vi "Drive Controller.vi"(8 "error in":errorcluster) -> ()   [LabVIEW 2019]
doc: "This VI executes continuously carrying out the current operation and responding to updates or new operation requests. It will often contain the timing or control code that is difficult to place directly in TeleOp. This VI generally opens all sensors and motors and isolates the rest of the robot code from knowing implementation details of how the operations are carried out."
uses:
  <vilib>/Rock Robotics/WPI/Framework/Completion Status.ctl
  Drive Setpoints.ctl
  Drive Operations.ctl
  <vilib>/Rock Robotics/WPI/SafetyOutput/WPI_SafetyOutputConfigMenu.ctl
  <vilib>/Rock Robotics/WPI/RobotDrive/WPI_RobotDriveOpen4MotorWithExistingMotors.vi
  <vilib>/Rock Robotics/WPI/RobotDrive/WPI_RobotDriveOpen2MotorWithTalon.vi
panel:
  in  "Interactive Values":T1
  in  "Buttons":cluster{"Execute Cmd":bool, "Abort Cmd":bool}
  out "Command Timing":cluster{"Start Time (ms)":u32, "Iterations":i32}
  out "Status":T3
  out "Setpoints":T4(graph)
  out "Current\nCmd":string
  # "Tip: The graph shows the motor setpoints. It may also be helpful to observe inputs and sensor values.\nYou may also want to display tuning or debugging controls."
  # "Interactive Command: You may fill in the settings for a command\nand schedule it with the Execute button. You can observe and abort\nany command while fine tuning the code for the controller."
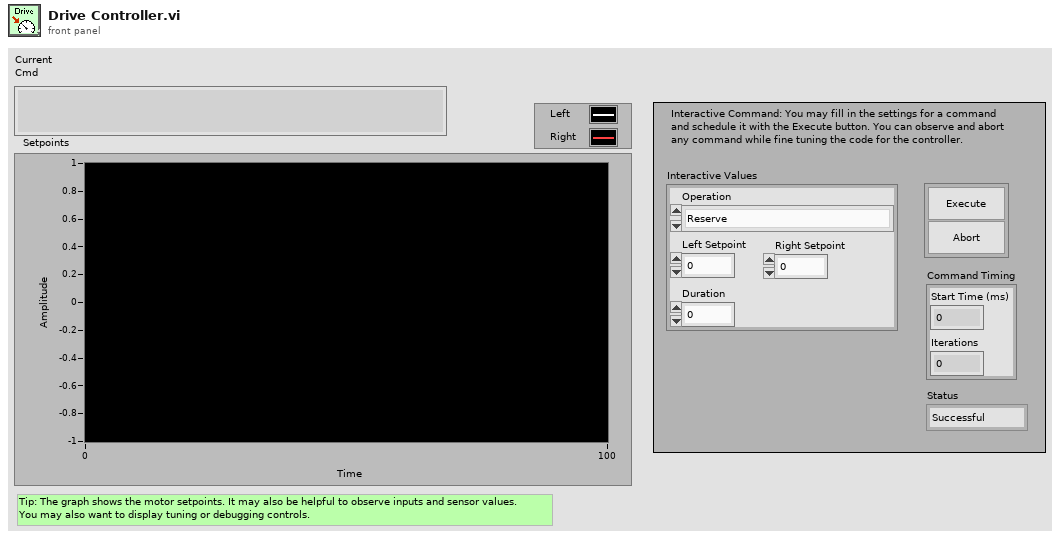
[diagram p1: front panel]
types:
  T1 = typedef "Drive Setpoints.ctl" = cluster{"Operation":T2, "Left Setpoint":dbl, "Right Setpoint":dbl, "Duration":dbl}
  T2 = typedef "Drive Operations.ctl" = enum16{"Reserve", "Read Current", "Immediate", "Drive for Time", "Drive for Distance"}
  T3 = typedef "Completion Status.ctl" = enum16{"Successful", "Aborted", "Incomplete"}
  T4 = cluster{"Left Setpoint":dbl, "Right Setpoint":dbl}
  T5 = typedef "WPI_SafetyOutputConfigMenu.ctl" = enum16{"Enable", "Disable"}
  T6 = typedef "WPI_RobotDriveDevRef.ctl" = cluster{"DevStatus":errorcluster, "Motors[]":T7[], "Square Inputs":bool, "Max Output":dbl}
  T7 = typedef "WPI_MotorControlDeviceRef.ctl" = cluster{"DeviceStatus":errorcluster, "Type":T8, "PWM":cluster{"PWM Channel":T9, "DeadBand":T10}, "CAN":cluster{"Device Number":u8, "SetOutput VI Ref":variant, "GetOutput VI Ref":variant, "Enable VI Ref":variant, "Disable VI Ref":variant, "Data":variant}, "Invert":bool, "DIO PWM":cluster{"PWM \"Enable\" Channel":T9, "DIOChannel":T11, "PWM Rate":dbl}}
  T8 = typedef "WPI_MotorControlType.ctl" = enum16{"PWM", "CAN", "DIO PWM"}
  T9 = typedef "FPGA_DIOPWMChannel.ctl" = enum8{"PWM 0", "PWM 1", "PWM 2", "PWM 3", "PWM 4", "PWM 5", "PWM 6", "PWM 7", "PWM 8", "PWM 9", "PWM MXP 0", "PWM MXP 1", "PWM MXP 2", "PWM MXP 3", "PWM MXP 4", "PWM MXP 5", "PWM MXP 6", "PWM MXP 7", "PWM MXP 8", "PWM MXP 9", "Invalid"}
  T10 = typedef "WPI_PWMDeadband.ctl" = cluster{"Name":string, "maxPositivePwm":i32, "minPositivePwm":i32, "centerPwm":i32, "maxNegativePwm":i32, "minNegativePwm":i32, "angularRange":u16}
  T11 = typedef "FPGA_DIOChannel.ctl" = enum8{"DIO 0", "DIO 1", "DIO 2", "DIO 3", "DIO 4", "DIO 5", "DIO 6", "DIO 7", "DIO 8", "DIO 9", "DIO MXP 0", "DIO MXP 1", "DIO MXP 2", "DIO MXP 3", "DIO MXP 4", "DIO MXP 5", "DIO MXP 6", "DIO MXP 7", "DIO MXP 8", "DIO MXP 9", "DIO MXP 10", "DIO MXP 11", "DIO MXP 12", "DIO MXP 13", "DIO MXP 14", "DIO MXP 15", "SPI Port CS1", "SPI Port CS2", "SPI Port CS3", "SPI Port MISO", "SPI Port MOSI", "Invalid"}
  T12 = typedef "Command Status Info.ctl" = cluster{"Name":string, "Status":T3, "notifier out":T13}
  T13 = typedef "Completion Notifier.ctl" = refnum<notifier>
  T14 = cluster{"SubSystem Data":T1, cluster{"Start Time (ms)":u32, "Iterations":i32}, cluster{"Command Info":T12, "Description":string, "Default Command":T1, "queue out":refnum<queue>, "Subsystem Name":string}}
  T15 = cluster{"SubSystem Data":T1, cluster{"Start Time (ms)":u32, "Iterations":i32}, "Default Command Arguments":cluster{"Command Info":T12, "Description":string, "Default Command":T1, "queue out":refnum<queue>, "Subsystem Name":string}}
  T16 = cluster{"Don't move motors while reserved":dbl, "Don't move motors while reserved":dbl}
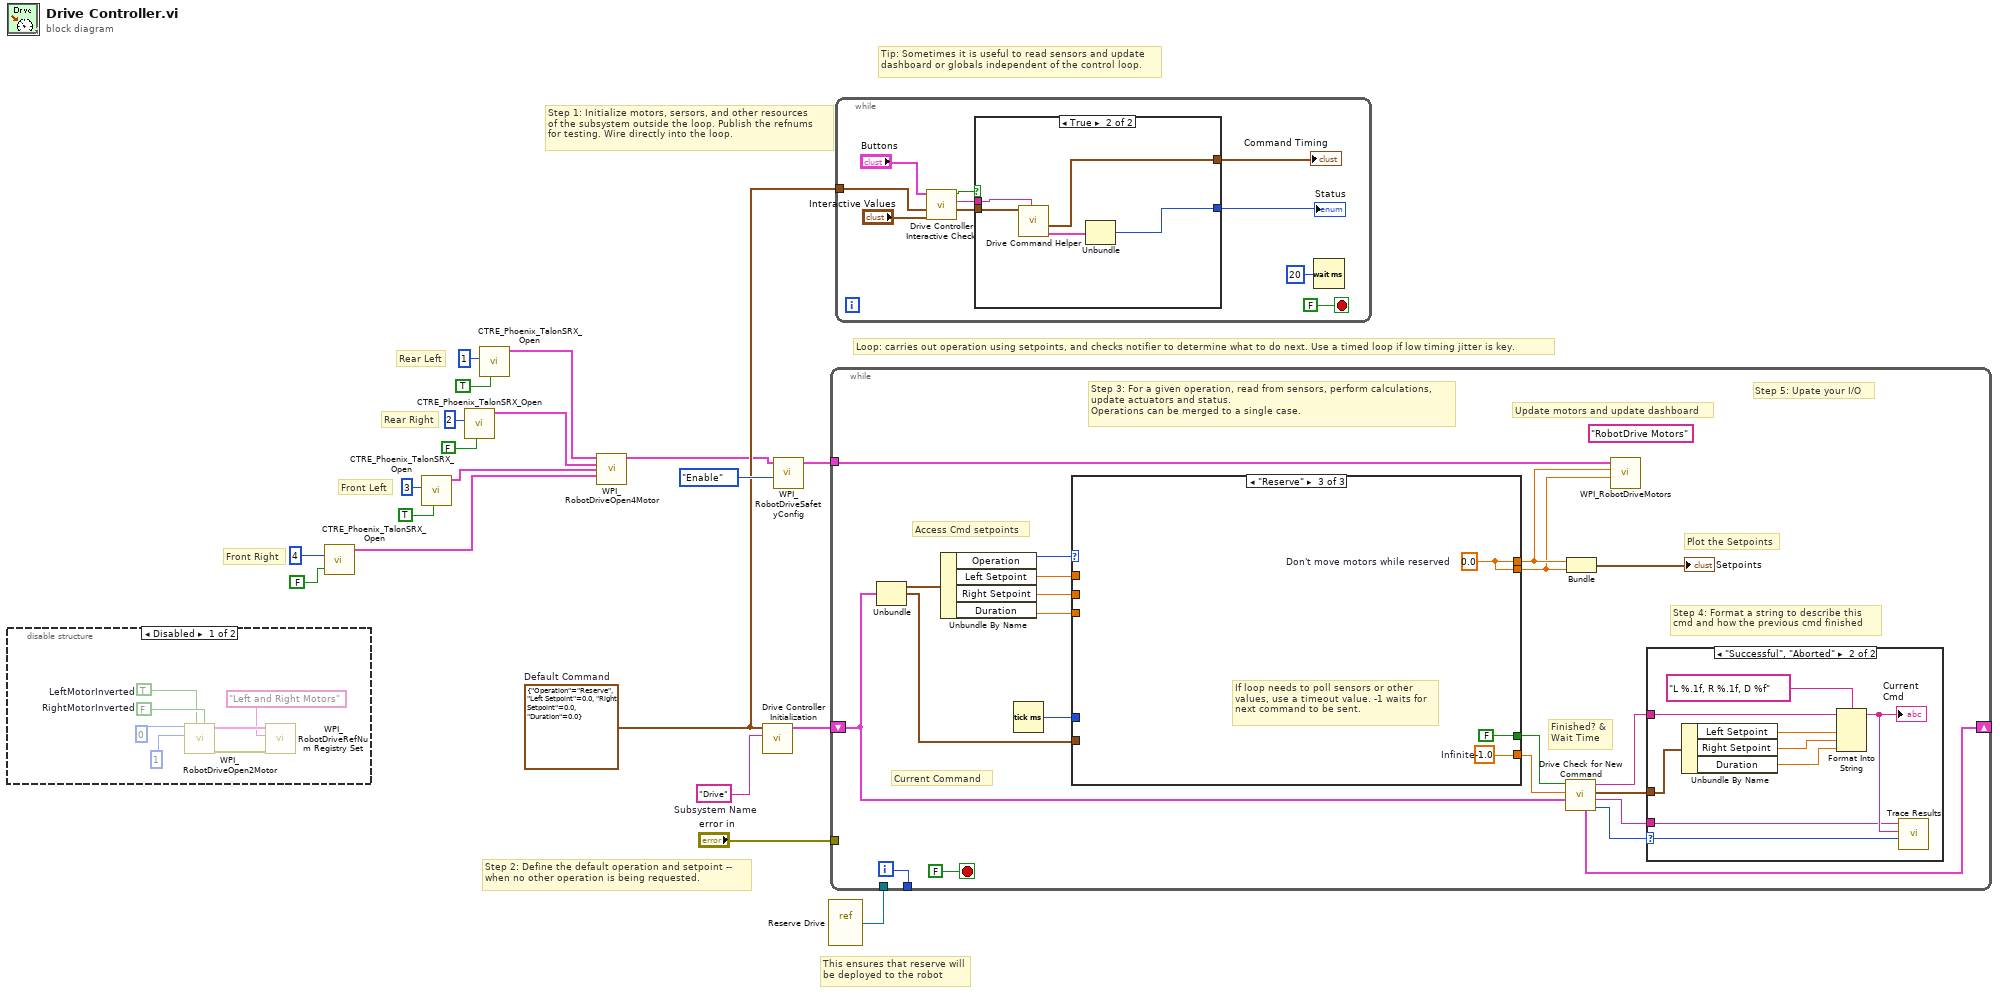
[diagram p0: block diagram]
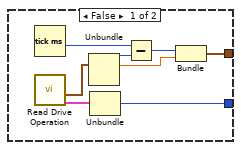
[diagram p3: hidden frame]
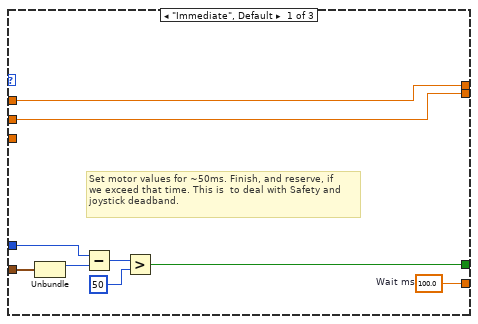
[diagram p5: hidden frame]
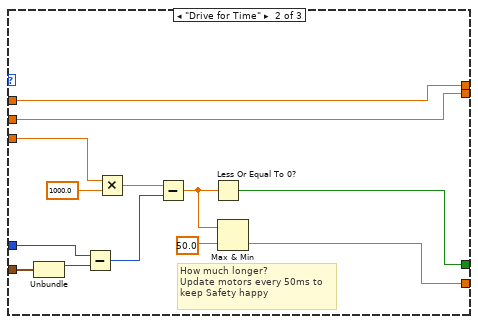
[diagram p6: hidden frame]
diagram:
  w14 = T1 {"Operation"=enum."Reserve", "Left Setpoint"=0.0, "Right Setpoint"=0.0, "Duration"=0.0}  # Default Command
  w20 = "Drive"  # Subsystem Name
  # "Front Right"
  # "Front Left"
  # "Rear Right"
  # "Rear Left"
  # "This ensures that reserve will\nbe deployed to the robot"
  # "Tip: Sometimes it is useful to read sensors and update\ndashboard or globals independent of the control loop."
  # "Step 2: Define the default operation and setpoint --\nwhen no other operation is being requested."
  # "Step 1: Initialize motors, sersors, and other resources\nof the subsystem outside the loop. Publish the refnums\nfor testing. Wire directly into the loop."
  # "Loop: carries out operation using setpoints, and checks notifier to determine what to do next. Use a timed loop if low timing jitter is key."
  n1 = disable-structure shown="Disabled" {
    frame Disabled {
      w24 = TRUE  # LeftMotorInverted
      w25 = FALSE  # RightMotorInverted
      n2 = call-poly <vilib>:"WPI_RobotDriveOpen2Motor.vi"("Right Motor Inverted"=w25, "Left Motor Inverted"=w24, "Right Motor"=u8 1 ("Left Motor"), "Left Motor"=u8 0) -> ("error out"=w21:errorcluster, "RobotDriveDevRef"=w23:T6)  [unwired: 1 in, 5 out]
      n3 = call <vilib>:"WPI_RobotDriveRefNum Registry Set.vi"("error in (no error)"=w21, "refnum name"="Left and Right Motors", "RobotDriveDevRef"=w23) -> ()  [unwired: 1 in, 8 out]
    }
    frame Enabled {
    }
  }
  n4 = call <vilib>:"CTRE_Phoenix_TalonSRX_Open.vi"("Invert"=FALSE, "Device Number"=u8 4) -> ("CAN Talon SRX Ref"=w2:T7)  [unwired: 8 in, 1 out]
  n5 = call <vilib>:"CTRE_Phoenix_TalonSRX_Open.vi"("Invert"=TRUE, "Device Number"=u8 3) -> ("CAN Talon SRX Ref"=w3:T7)  [unwired: 8 in, 1 out]
  n6 = call <vilib>:"CTRE_Phoenix_TalonSRX_Open.vi"("Invert"=FALSE, "Device Number"=u8 2) -> ("CAN Talon SRX Ref"=w4:T7)  [unwired: 8 in, 1 out]
  n7 = call <vilib>:"CTRE_Phoenix_TalonSRX_Open.vi"("Invert"=TRUE, "Device Number"=u8 1) -> ("CAN Talon SRX Ref"=w5:T7)  [unwired: 8 in, 1 out]
  n8 = call-poly <vilib>:"WPI_RobotDriveOpen4Motor.vi"("Rear Left Motor Dev Ref"=w5, "Rear Right Motor Dev Ref"=w4, "Front Left Motor Dev Ref"=w3, "Front Right Motor Dev Ref"=w2) -> ("RobotDriveDevRef"=w1:T6)  [unwired: 10 in, 1 out]
  n9 = call "Drive Controller Initialization.vi"("Subsystem Name"=w20, "Default Command"=w14) -> ("Current Command"=w16:T14)  [unwired: 9 in]
  n10 = call <vilib>:"WPI_RobotDriveSafetyConfig.vi"("mode"=WPI_SafetyOutputConfigMenu."Enable", "RobotDriveDevRef"=w1) -> ("RobotDriveDevRef"=w18:T6)  [unwired: 8 in, 1 out]
  n11 = vi-ref "Reserve Drive.vi"() -> (w15:refnum<vi>)
  n12 = while {
    shift-right: [w35] -> _
    shift-left: w16 -> [w28]
    tunnel: [w47] -> _
    tunnel: w18 -> [w43]
    tunnel: "error in" -> [_]
    tunnel: w15 -> [_]
    i -> [w47]
    stop <- FALSE stop-if-true
    (unwired) "RobotDrive Motors" ("Name")
    # "Step 5: Upate your I/O"
    # "Step 4: Format a string to describe this\ncmd and how the previous cmd finished"
    # "Current Command"
    # "Update motors and update dashboard"
    # "Plot the Setpoints"
    # "Access Cmd setpoints"
    # "Finished? &\nWait Time"
    # "Step 3: For a given operation, read from sensors, perform calculations,\nupdate actuators and status.\nOperations can be merged to a single case."
    n13 = Unbundle(w28) -> ("SubSystem Data"=w42:T1, w29:cluster{"Start Time (ms)":u32, "Iterations":i32})  [unwired: 1 out]
    n14 = Unbundle By Name(w42) -> ("Operation"=w41:T2, "Left Setpoint"=w40:dbl, "Right Setpoint"=w39:dbl, "Duration"=w38:dbl)
    n15 = Tick Count (ms)() -> (millisecond timer value=w37:u32)
    n16 = case shown="\"Reserve\"" w41 {
      tunnel: [w66 w67 w82] -> w34
      tunnel: [w59 w74 FALSE ("ignore previous (F)")] -> w33
      tunnel: w29 -> [w58 w76 _]
      tunnel: [w65 w73 w80] -> w45
      tunnel: [w64 w72 w80] -> w44
      tunnel: w40 -> [w65 w73 _]
      tunnel: w39 -> [w64 w72 _]
      tunnel: w38 -> [_ w71 _]
      tunnel: w37 -> [w60 w70 _]
      frame "Immediate", Default {
        w66 = 100.0  # Wait ms
        # "Set motor values for ~50ms. Finish, and reserve, if\nwe exceed that time. This is  to deal with Safety and\njoystick deadband."
        n17 = Unbundle(w58) -> ("Start Time (ms)"=w61:u32)  [unwired: 1 out]
        n18 = Subtract(x=w60, y=w61) -> (x-y=w62:u32)
        n19 = Greater?(x=w62, y=u8 50 ("Left Motor")) -> (0:w59:bool)
      }
      frame "Drive for Time" {
        # "How much longer?\nUpdate motors every 50ms to\nkeep Safety happy"
        n20 = Unbundle(w76) -> ("Start Time (ms)"=w75:u32)  [unwired: 1 out]
        n21 = Subtract(x=w70, y=w75) -> (x-y=w79:u32)
        n22 = Multiply(x=w71, y=1000.0) -> (x*y=w78:dbl)
        n23 = Subtract(x=w78, y=w79) -> (x-y=w69:dbl)
        n24 = Less Or Equal To 0?(x=w69) -> (x <= 0?=w74:bool)
        n25 = Max & Min(x=w69, y=50.0) -> (min(x,y)=w67:dbl)  [unwired: 1 out]
      }
      frame "Reserve" {
        w80 = 0.0  # Don't move motors while reserved
        w82 = -1.0  # Infinite
        # "If loop needs to poll sensors or other\nvalues, use a timeout value. -1 waits for\nnext command to be sent."
      }
    }
    n26 = call "Drive Check for New Command.vi"("input cluster"=w28, "Wait time (ms)"=w34, "Finished?"=w33) -> ("Completion"=w36:T3, "Subsystem Name"=w30:string, "Current Command"=w31:T1, "Initial Trace String"=w32:string, "Next Command"=w35:T15)  [unwired: 4 in]
    n27 = Bundle("Don't move motors while reserved"=w45, "Don't move motors while reserved"=w44) -> (→"Setpoints":T16)  [unwired: 1 in]
    n28 = call <vilib>:"WPI_RobotDriveMotors.vi"("RightSpeed"=w44, "LeftSpeed"=w45, "RobotDriveDevRef"=w43) -> ()  [unwired: 1 in, 8 out]
    n29 = case shown="\"Successful\", \"Aborted\"" w36 {
      selector: w36 -> [_ w57]
      tunnel: w32 -> [_ w52]
      tunnel: w31 -> [_ w53]
      tunnel: w30 -> [_ w49]
      frame "Incomplete", Default {
        # "Continuing current command"
      }
      frame "Successful", "Aborted" {
        # "Report and setup for next command"
        n30 = Unbundle By Name(w53) -> ("Left Setpoint"=w55:dbl, "Right Setpoint"=w56:dbl, "Duration"=w50:dbl)
        n31 = Format Into String(format string="L %.1f, R %.1f, D %f", initial string=w52, w55, w56, w50) -> (resulting string=w51:string)  [unwired: 1 in, 1 out]
        "Current\nCmd" <- w51
        n32 = call <vilib>:"Trace Results.vi"("Status of previous command"=w57, "Description"=w51, "Subsystem"=w49) -> ()  [unwired: 9 in]
      }
    }
  }
  n33 = while {
    tunnel: w14 -> [w84]
    stop <- FALSE stop-if-true
    n34 = call "Drive Controller Interactive Check.vi"("Interactive Command In"="Interactive Values", "Default Command"=w84, "Buttons"="Buttons") -> ("Interactive Command Out"=w86:T1, "Trace String"=w87:string, "Schedule"=w88:bool)  [unwired: 6 in]
    n35 = case shown="True" w88 {
      tunnel: [w97 w105] -> w89
      tunnel: [w96 w101] -> w90
      tunnel: w87 -> [_ w103]
      tunnel: w86 -> [_ w102]
      frame False {
        n36 = Tick Count (ms)() -> (millisecond timer value=w100:u32)
        n37 = call "Read Drive Operation.vi"() -> ("Command Info"=w94:T12, "SubSystem Data"=w93:T1)  [unwired: 9 in, 1 out]
        n38 = Unbundle(w93) -> ("Operation"=w98:T2, "Left Setpoint"=w95:dbl)  [unwired: 2 out]
        n39 = Unbundle(w94) -> ("Status"=w97:T3)  [unwired: 2 out]
        n40 = Subtract(x=w100, y=w98) -> (x-y=w99:u32)
        n41 = Bundle(w99, "Left Setpoint"=w95) -> (w96:cluster{u32, "Left Setpoint":dbl})  [unwired: 1 in]
      }
      frame True {
        n42 = call "Drive Command Helper.vi"("Description"=w103, "SubSystem Data"=w102) -> ("Command Info Out"=w104:T12, "Command Timing"=w101:cluster{"Start Time (ms)":u32, "Iterations":i32})  [unwired: 7 in, 1 out]
        n43 = Unbundle(w104) -> ("Status"=w105:T3)  [unwired: 2 out]
      }
    }
    "Status" <- w89
    "Command Timing" <- w90
    n44 = Wait (ms)(milliseconds to wait=u32 20) -> ()  [unwired: 1 out]
  }
